vi "湿度自动滚条.vi"(0 "湿度输入1":dbl, 1 "移位输入1":string[][](array[string]), 5 "湿度输入 2":dbl, 7 "循环计数":dbl, 9 "历史最高":dbl, 11 "历史最低":dbl, 12 "移位输入2":dbl, 13 "行数":dbl) -> (4 "移位输出1":string[][](array[string]), 6 "移位输出2":dbl, 8 "表格输出":string[][](table), 10 "湿度簇":T1, 15 "簇输出":T2 caption="输出簇")   [LabVIEW 2012]
uses:
  <vilib>/Utility/miscctls.llb/LVRowAndColumnUnsignedTypeDef.ctl
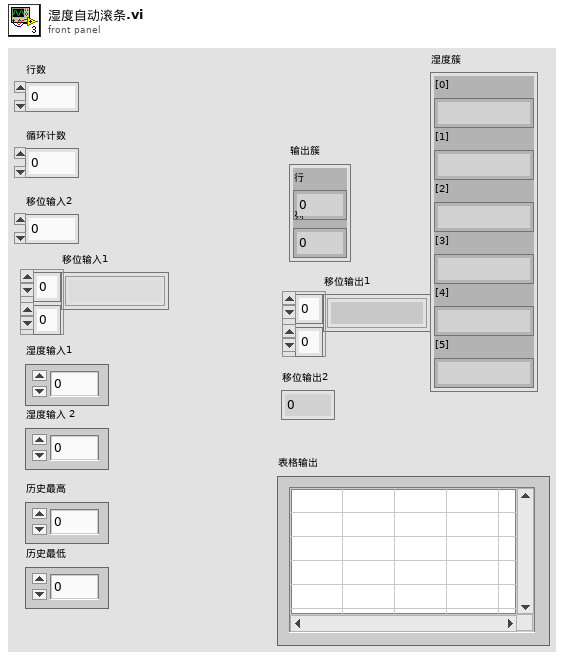
[diagram p1: front panel]
types:
  T1 = cluster{"[0]":string, "[1]":string, "[2]":string, "[3]":string, "[4]":string, "[5]":string}
  T2 = typedef "LVRowAndColumnUnsignedTypeDef.ctl" = cluster{"Row":u32, "Column":u32}
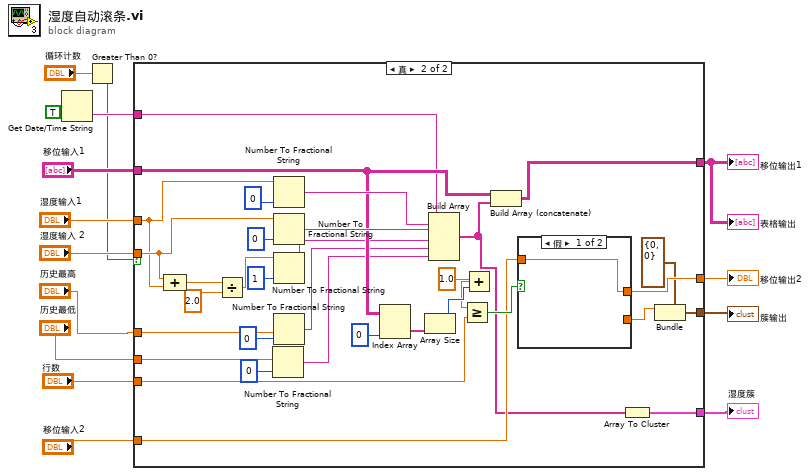
[diagram p0: block diagram]
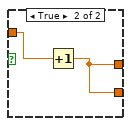
[diagram p3: hidden frame]
diagram:
  n1 = Get Date/Time String(want seconds? (F)=TRUE ("需要秒？(F)")) -> (time string=w5:string)  [unwired: 2 in, 1 out]
  n2 = Greater Than 0?(x="循环计数") -> (x > 0?=w2:bool)
  n3 = case shown="真" w2 {
    tunnel: [_ w44] -> w15
    tunnel: "历史最高" -> [_ w39]
    tunnel: "湿度输入 2" -> [_ w26]
    tunnel: "移位输入2" -> [_ w38]
    tunnel: "移位输入1" -> [_ w37]
    tunnel: [_ w35] -> w10
    tunnel: [_ w34] -> w9
    tunnel: "行数" -> [_ w33]
    tunnel: "湿度输入1" -> [_ w25]
    tunnel: w5 -> [_ w32]
    tunnel: "历史最低" -> [_ w31]
    tunnel: [_ w16] -> w1
    frame False {
    }
    frame True {
      n4 = Compound Arithmetic op=ADD(w26, w25) -> (w24:dbl)
      n5 = Divide(x=w24, y=2.0) -> (x/y=w22:dbl)
      n6 = Number To Fractional String(number=w31, precision (6)=i16 0 ("精度(6)")) -> (F-format string=w19:string)  [unwired: 2 in]
      n7 = Number To Fractional String(number=w25, precision (6)=i16 0 ("精度(6)")) -> (F-format string=w42:string)  [unwired: 2 in]
      n8 = Number To Fractional String(number=w26, precision (6)=i16 0 ("精度(6)")) -> (F-format string=w40:string)  [unwired: 2 in]
      n9 = Number To Fractional String(number=w22, precision (6)=i16 1 ("精度(6)")) -> (F-format string=w21:string)  [unwired: 2 in]
      n10 = Number To Fractional String(number=w39, precision (6)=i16 0 ("精度(6)")) -> (F-format string=w20:string)  [unwired: 2 in]
      n11 = Index Array(array=w37, index (col)=0 ("索引")) -> (element=w49:string[])  [unwired: 1 in]
      n12 = Array Size(array=w49) -> (size(s)=w47:i32)
      n13 = Build Array(w32, w42, w40, w21, w20, w19) -> (w17:string[])
      n14 = Add(x=1.0, y=w47) -> (x+y=w46:dbl)
      n15 = Greater Or Equal?(x=w46, y=w33) -> (x >= y?=w45:bool)
      n16 = Build Array (concatenate)(w37, w17) -> (w35:string[][])
      n17 = case shown="假" w45 {
        tunnel: w38 -> [w50 w51]
        tunnel: [w50 w52] -> w44
        tunnel: [_ w52] -> w43
        frame False {
        }
        frame True {
          n18 = Increment(x=w51) -> (x+1=w52:dbl)
        }
      }
      n19 = Array To Cluster(array=w17) -> (cluster=w16:T1)
      n20 = Bundle(cluster=T2 {"Row"=0, "Column"=0} ("索引值"), "Row"=w43) -> (w34:T2)  [unwired: 1 in]
    }
  }
  "移位输出2" <- w15
  "移位输出1" <- w10
  "表格输出" <- w10
  "簇输出" <- w9
  "湿度簇" <- w1
